vi "test_cvi.vi"() -> ()   [LabVIEW 2015]
panel:
  out "XY Graph":cluster{"lags":dbl[], "acf":dbl[]}(graph)
  out "lags":dbl[](array[numeric])
  in  "offset_lag":dbl
  in  "coarseness":dbl=8.0
  in  "stop_time_ps":dbl=100000000000000.0
  in  "start_time_ps":dbl=10000000.0
  in  "error in (no error)":errorcluster
  out "times":dbl[](array[numeric])
  in  "tmode":u8=2
  in  "device":u8
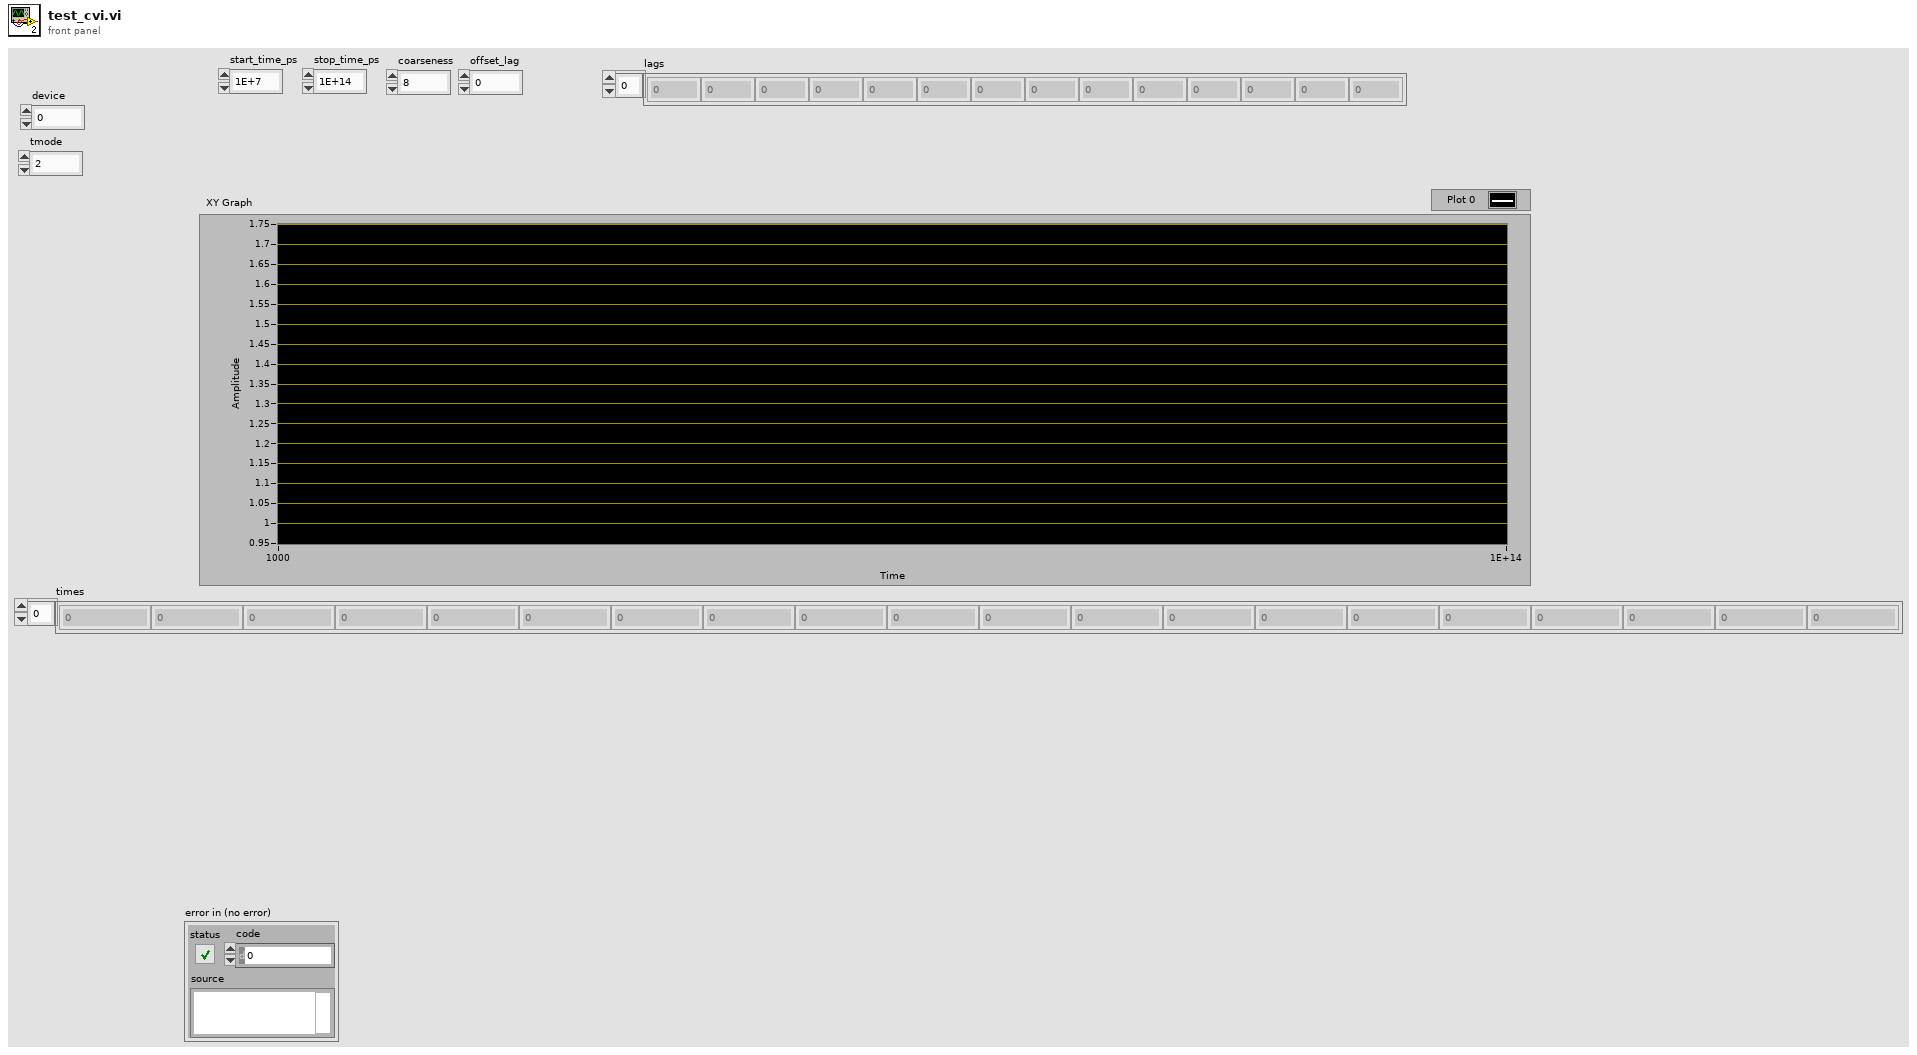
[diagram p1: front panel]
types:
  T1 = enum16{"big-endian, network order", "native, host order", "little-endian"}
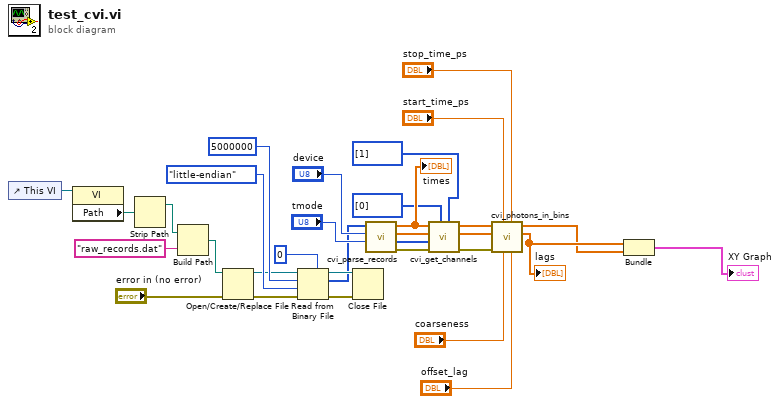
[diagram p0: block diagram]
diagram:
  n1 = control-ref of="This VI"() -> (w27:refnum<vi>)
  n2 = property class="VI"(reference=w27) -> ("Path"=w28:path)  [unwired: 1 in, 2 out]
  n3 = Strip Path(path=w28) -> (stripped path=w18:path)  [unwired: 1 out]
  n4 = Build Path(base path=w18, name or relative path="raw_records.dat") -> (appended path=w30:path)
  n5 = Open/Create/Replace File(file path (use dialog)=w30, error in="error in (no error)") -> (refnum out=w19:refnum<file>, error out=w20:errorcluster)  [unwired: 4 in, 1 out]
  n6 = Read from Binary File(5:u32 0, 8:w20, 9:T1."little-endian" ("byte order (0:big-endian, network order)"), 10:5000000 ("count (1)"), 11:w19) -> (0:w22:errorcluster, 2:w17:u32[], 3:w21:refnum<file>)  [unwired: 1 in, 1 out]
  n7 = Close File(refnum=w21, error in=w22) -> ()  [unwired: 2 out]
  n8 = call "cvi_parse_records.vi"("tmode"="tmode", "device"="device", "fifo_buffer"=w17) -> ("error out"=w8:errorcluster, "channels"=w14:u8[], "sync"=w15:dbl[], "times"=w16:dbl[])  [unwired: 5 in]
  "times" <- w16
  n9 = call "cvi_get_channels.vi"("arm2_channels"=u8[] [1], "arm1_channels"=u8[] [0], "error in (no error)"=w8, "channels"=w14, "sync"=w15, "times"=w16) -> ("error out"=w9:errorcluster, "arm2"=w10:dbl[], "arm1"=w11:dbl[])  [unwired: 3 in]
  n10 = call "cvi_photons_in_bins.vi"("offset_lag"="offset_lag", "stop_time_ps"="stop_time_ps", "coarseness"="coarseness", "start_time_ps"="start_time_ps", "error in (no error)"=w9, "ch2"=w10, "ch1"=w11) -> ("lags"=w3:dbl[], "acf"=w2:dbl[])  [unwired: 2 in, 1 out]
  "lags" <- w3
  n11 = Bundle("lags"=w3, "acf"=w2) -> (→"XY Graph":cluster{"lags":dbl[], "acf":dbl[]})  [unwired: 1 in]
